vi "Read Assert.vi"(6 "Register with caller test (F)":bool, 7 "Assert Only? (F)":bool, 8 "error in (no error)":errorcluster, 10 "VI Call Chain":string[](array[string]), 11 "Assert Factory in":refnum<class "Test Assert Factory.lvclass">) -> (0 "error out":errorcluster, 2 "Assert":refnum<class "Assert.lvclass">, 3 "Assert Factory out":refnum<class "Test Assert Factory.lvclass">)   [LabVIEW 2013, in "Caraya.lvlib" / "Test Assert Factory.lvclass"]
doc: "Returns the Assert implementation being used for a specific VI."
uses:
  Test Assert Factory.lvclass
  Assert/Assert.lvclass
  Assert/Assert.lvclass/Assert.ctl
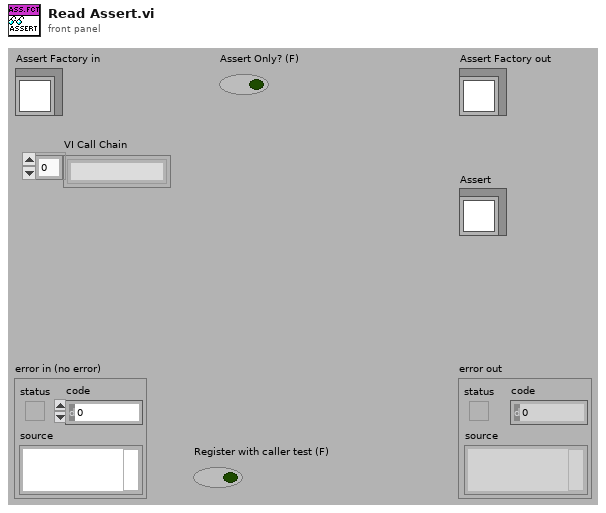
[diagram p1: front panel]
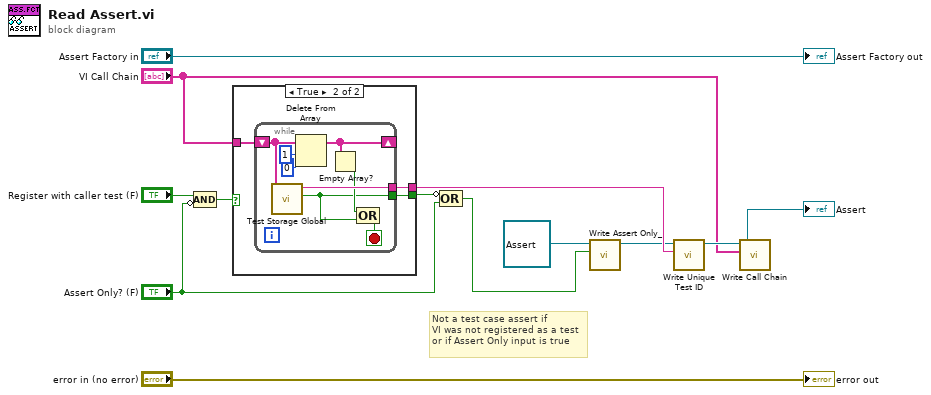
[diagram p0: block diagram]
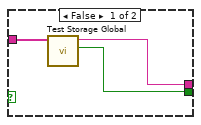
[diagram p2: hidden frame]
diagram:
  # "Not a test case assert if\nVI was not registered as a test\nor if Assert Only input is true"
  n1 = Compound Arithmetic op=AND("Register with caller test (F)", invert "Assert Only? (F)") -> (w1:bool)
  n2 = case shown="True" w1 {
    tunnel: [w14 w19] -> w11
    tunnel: [w16 w18] -> w9
    tunnel: "VI Call Chain" -> [w15 w17]
    frame False {
      n3 = call "Test Storage Global.vi"("VI Call Chain"=w15) -> ("Found/Replaced?"=w14:bool, "Unique Test ID"=w16:string)  [unwired: 7 in, 2 out]
    }
    frame True {
      n4 = while {
        tunnel: [w25] -> w19
        tunnel: [w27] -> w18
        shift-right: [w22] -> _
        shift-left: w17 -> [w23]
        stop <- w24 stop-if-true
        n5 = call "Test Storage Global.vi"("VI Call Chain"=w23) -> ("Found/Replaced?"=w25:bool, "Unique Test ID"=w27:string)  [unwired: 7 in, 2 out]
        n6 = Delete From Array(array=w23, length=1, index=0) -> (array with subset deleted=w22:string[])  [unwired: 1 out]
        n7 = Empty Array?(array=w22) -> (empty?=w26:bool)
        n8 = Compound Arithmetic op=OR(w26, w25) -> (w24:bool)
      }
    }
  }
  n9 = Compound Arithmetic op=OR(invert w11, "Assert Only? (F)") -> (w10:bool)
  n10 = call "Write Assert Only_.vi"("Assert Only?"=w10, "Assert"=refnum<class "Assert.lvclass"> refnum ("Caraya.lvlib:Assert.lvclass")) -> ("Assert"=w7:refnum<class "Assert.lvclass">)  [unwired: 8 in, 1 out]
  n11 = call "Write Unique Test ID.vi"("Unique Test ID"=w9, "Assert"=w7) -> ("Assert out"=w6:refnum<class "Assert.lvclass">)  [unwired: 9 in]
  n12 = call "Write Call Chain.vi"("Call Chain"="VI Call Chain", "Assert in"=w6) -> ("Assert out"=→"Assert":refnum<class "Assert.lvclass">)  [unwired: 9 in]
  "error out" <- "error in (no error)"
  "Assert Factory out" <- "Assert Factory in"
